vi "fftw_test.vi"() -> ()   [LabVIEW 2020]
uses:
  FFTWDLL.lvlib
panel:
  out "time per FFT [ms]":dbl
  in  "repeat":i32=1
  in  "Numeric":i32=256
  out "Y":cdb[](array[numeric])
  out "error out":errorcluster
  in  "error in (no error)":errorcluster
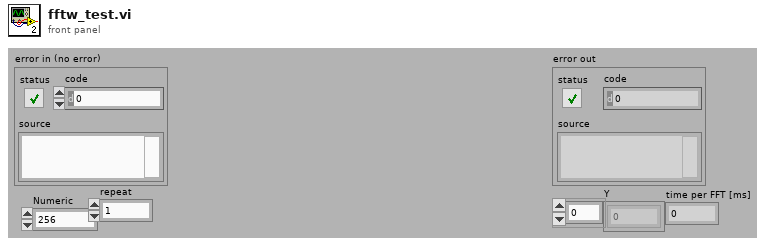
[diagram p1: front panel]
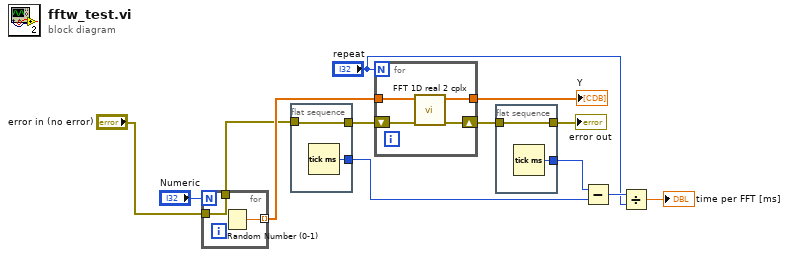
[diagram p0: block diagram]
diagram:
  n1 = for {
    N: "Numeric" -> [_]
    tunnel: [w15] -> w13 mode=indexing
    tunnel: "error in (no error)" -> [w14]
    tunnel: [w14] -> w8
    n2 = Random Number (0-1)() -> (number: 0 to 1=w15:dbl)
  }
  n3 = flat-sequence {
    tunnel: w8 -> [w17]
    tunnel: [w17] -> w9
    tunnel: [w16] -> w4
    frame #0 {
      n4 = Tick Count (ms)() -> (millisecond timer value=w16:u32)
    }
  }
  n5 = for {
    N: "repeat" -> [_]
    tunnel: w13 -> [w19]
    tunnel: [w18] -> w11
    shift-right: [w20] -> w7
    shift-left: w9 -> [w21]
    n6 = call "FFT 1D real 2 cplx.vi"("error in (no error)"=w21, "y"=w19) -> ("error out"=w20:errorcluster, "Y"=w18:cdb[])  [unwired: 6 in, 2 out]
  }
  "Y" <- w11
  n7 = flat-sequence {
    tunnel: w7 -> [w23]
    tunnel: [w23] -> w6
    tunnel: [w22] -> w5
    frame #0 {
      n8 = Tick Count (ms)() -> (millisecond timer value=w22:u32)
    }
  }
  n9 = Subtract(x=w5, y=w4) -> (x-y=w3:u32)
  n10 = Divide(x=w3, y="repeat") -> (x/y=→"time per FFT [ms]":dbl)
  "error out" <- w6
